vi "Boolean.vi"(8 "error in":errorcluster, 11 "GObj Refnum":refnum<vi>) -> (0 "error out":errorcluster, 3 "Boolean out":refnum<class "Boolean.lvclass">)   [LabVIEW 2014, in "Raspberry Pi Compatible Compiler for LabVIEW.lvlib" / "Boolean.lvclass"]
uses:
  Boolean.lvclass
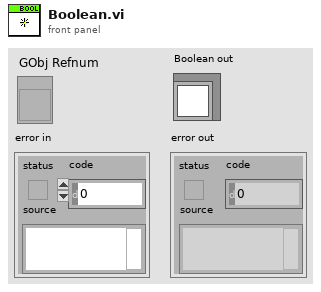
[diagram p1: front panel]
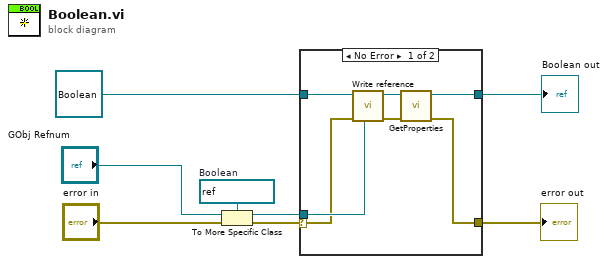
[diagram p0: block diagram]
diagram:
  w8 = refnum<vi> refnum  # Boolean
  n1 = To More Specific Class(target class=w8, reference="GObj Refnum", error in="error in") -> (specific class reference=w6:refnum<vi>, error out=w7:errorcluster)
  n2 = case shown="No Error" w7 {
    selector: w7 -> [w12 w17]
    tunnel: refnum<class "Boolean.lvclass"> refnum ("Boolean in") -> [w15 w16]
    tunnel: w6 -> [w13 _]
    tunnel: [w10 w16] -> w4
    tunnel: [w9 w17] -> w3
    frame No Error {
      n3 = call-dynamic "Write reference.vi"("reference"=w13, "error in"=w12, "GObject in"=w15) -> ("error out"=w11:errorcluster, "GObject out"=w14:refnum<class "Boolean.lvclass">)  [unwired: 5 in]
      n4 = call-dynamic "GetProperties.vi"("error in"=w11, "Boolean in"=w14) -> ("error out"=w9:errorcluster, "Boolean out"=w10:refnum<class "Boolean.lvclass">)  [unwired: 8 in]
    }
    frame Error {
    }
  }
  "error out" <- w3
  "Boolean out" <- w4
